vi "Standby Power Stats.vi"(8 "Error In":errorcluster, 11 "Full Data Array":dbl[](array[numeric])) -> (0 "Error Out":errorcluster, 1 "Power Variation (%)":dbl, 2 "Maximum Power (Watts)":dbl, 3 "Standby Power - Pia (Watts)":dbl)   [LabVIEW 2020]
uses:
  <vilib>/Analysis/baseanly.llb/Mean (DBL).vi
  <vilib>/Analysis/NI_AALBase.lvlib
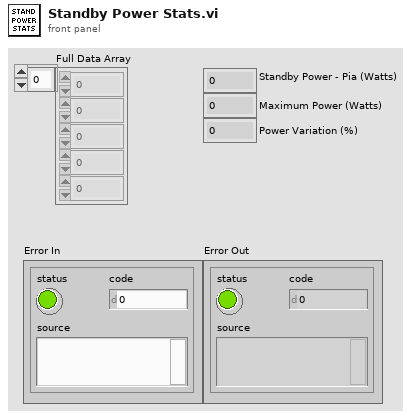
[diagram p1: front panel]
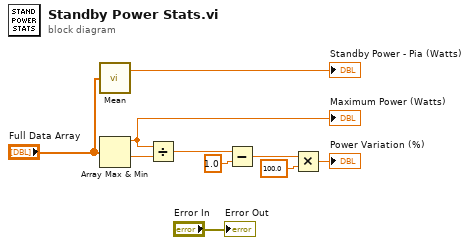
[diagram p0: block diagram]
diagram:
  n1 = call-poly <vilib>:"Mean.vi"("X"="Full Data Array") -> ("mean"=→"Standby Power - Pia (Watts)":dbl)  [unwired: 1 out]
  n2 = Array Max & Min(array="Full Data Array") -> (max value=w8:dbl, min value=w2:dbl)  [unwired: 2 out]
  "Maximum Power (Watts)" <- w8
  n3 = Divide(x=w8, y=w2) -> (x/y=w3:dbl)
  n4 = Subtract(x=w3, y=1.0) -> (x-y=w5:dbl)
  n5 = Multiply(x=w5, y=100.0) -> (x*y=→"Power Variation (%)":dbl)
  "Error Out" <- "Error In"
